vi "PXI O2 Sensor sim.vi"() -> ()   [LabVIEW 2014]
uses:
  <vilib>/eio/EIONode/EIONode.xnode
  <vilib>/rvi/eio/common/nirviEmuTemplateMethod_errors.vi
  <vilib>/NI Veristand/FPGA/NI_VS FPGA Support.lvlib
panel:
  in  "offset error":fxp<+/-,20,5>
  out "Connector0/AI1":i16
  in  "PWM measurement timeout":u32=40000
  out "High time":u32
  out "Low Time":u32
  in  "heater voltage threshold":i16=1500
  in  "negate input?":bool
  out "Iteration time (ticks)":u32
  in  "Period (ticks)":u32=400
  in  "scaled coefficients":i32[](array[numeric])=[-270931504, 720512000, 156040332]
  in  "vBatt":fxp<+/-,16,5>=10.0
  out "Vn out":fxp<+/-,20,5>
  out "Ip. volts in":fxp<+/-,36,16>
  out "Ip":fxp<+/-,32,10> format="%^#_6e"
  in  "Lambda":fxp<+,12,3>=1.0
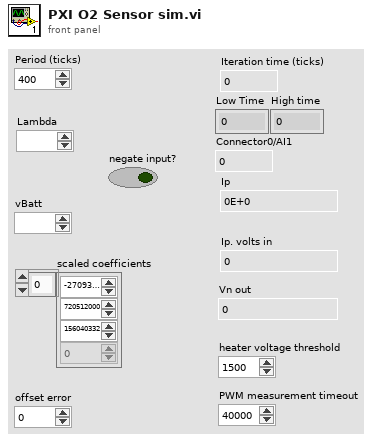
[diagram p1: front panel]
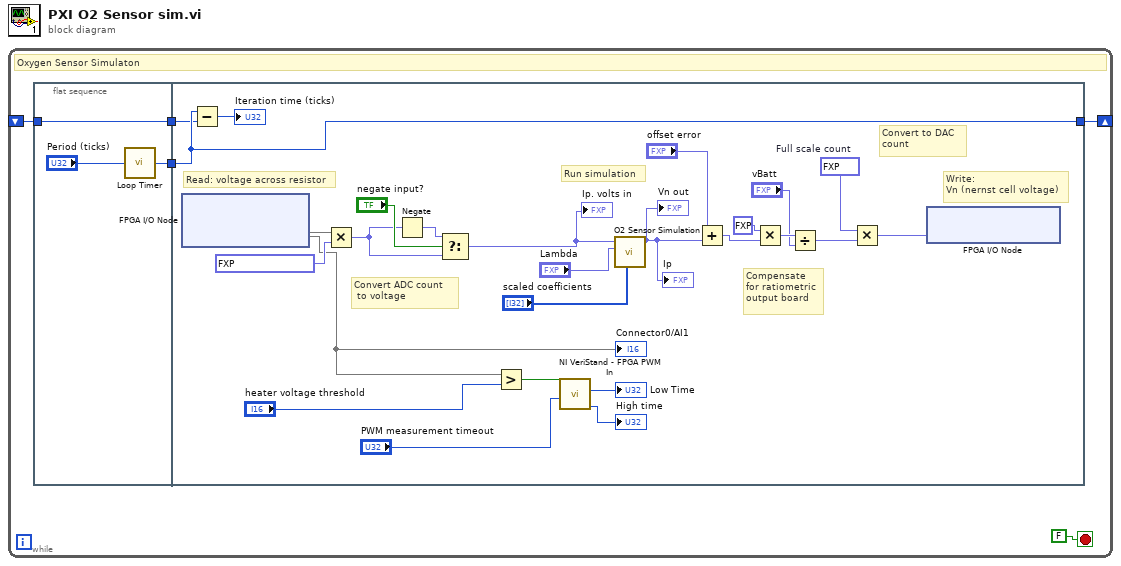
[diagram p0: block diagram]
diagram:
  n1 = while {
    shift-right: [w3] -> _
    shift-left: _ -> [w1]
    stop <- FALSE stop-if-true
    # "Oxygen Sensor Simulaton"
    n2 = flat-sequence {
      tunnel: [w7] -> w4
      tunnel: [w6] -> w2
      tunnel: w1 -> [w6]
      tunnel: w4 -> [w27]
      tunnel: [w27] -> w3
      tunnel: w2 -> [w26]
      frame #0 {
        n3 = call "Loop Timer"("Count(Ticks)"="Period (ticks)") -> ("Tick Count(Ticks)"=w7:u32)
      }
      frame #1 {
        w34 = fxp<+,16,15> 3276.5  # Full scale count
        # "Compensate\nfor ratiometric\noutput board"
        # "Convert to DAC\ncount"
        # "Convert ADC count\n to voltage"
        # "Run simulation"
        # "Write:\nVn (nernst cell voltage)"
        # "Read: voltage across resistor"
        n4 = xnode "FPGA I/O Node"() -> ("Connector0/AI0"=w23, "Connector0/AI1"=w16)  [unwired: 2 in, 2 out]
        "Connector0/AI1" <- w16
        n5 = Subtract(x=w27, y=w26) -> (x-y=→"Iteration time (ticks)":u32)
        n6 = Multiply(x=w23, y=fxp<+,20,0> 0.00030517578125 ("input conversion")) -> (x*y=w21:fxp<+,40,0>)
        n7 = Negate(x=w21) -> (-x=w22:fxp<+/-,41,1>)
        n8 = Select(t=w22, s="negate input?", f=w21) -> (s? t:f=w20:fxp<+/-,41,1>)
        "Ip. volts in" <- w20
        n9 = Greater?(x=w16, y="heater voltage threshold") -> (0:w17:bool)
        n10 = call <vilib>:"NI VeriStand - FPGA PWM In.vi"("Time Out"="PWM measurement timeout", "Value"=w17) -> ("High time"=→"High time":u32, "Low Time"=→"Low Time":u32)  [unwired: 8 out]
        n11 = call "O2 Sensor Simulation.vi"("scaled coefficients"="scaled coefficients", "Lambda"="Lambda", "Voltage at Ip in"=w20) -> ("Vn Out"=w11:fxp<+/-,20,5>)  [unwired: 7 in, 1 out]
        "Ip" <- w11
        "Vn out" <- w11
        n12 = Add(x="offset error", y=w11) -> (x+y=w10:fxp<+/-,21,6>)
        n13 = Multiply(x=fxp<+/-,20,5> 10.0, y=w10) -> (x*y=w31:fxp<+/-,41,11>)
        n14 = Divide(x=w31, y="vBatt") -> (x/y=w30:fxp<+/-,57,22>)
        n15 = Multiply(x=w34, y=w30) -> (x*y=w32:fxp<+/-,64,36>)
        n16 = xnode "FPGA I/O Node"("Connector0/AO0"=w32) -> ()  [unwired: 1 in, 1 out]
      }
    }
  }
